vi "Expand FIFO Type Def Release.vi"(7 "Control Refnum":refnum<vi>, 8 "error in (no error)":errorcluster, 10 "Array":refnum<vi>[](array[refnum]), 11 "Cluster in":refnum<vi>) -> (0 "error out":errorcluster)   [LabVIEW 2014, in "Initialization and IO Node Scripting.lvlib"]
uses:
  Initialization and IO Node Scripting.lvlib
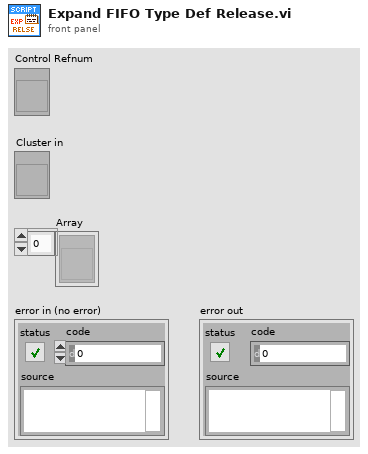
[diagram p1: front panel]
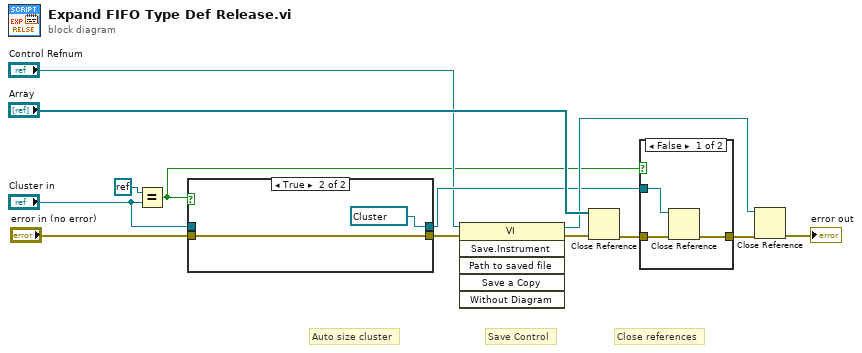
[diagram p0: block diagram]
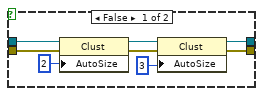
[diagram p3: hidden frame]
diagram:
  # "Auto size cluster"
  # "Save Control"
  # "Close references"
  n1 = Equal?(x=refnum<k0> refnum, y="Cluster in") -> (x = y?=w1:bool)
  n2 = case shown="True" w1 {
    tunnel: "error in (no error)" -> [w21 w23]
    tunnel: [w16 w23] -> w6
    tunnel: [w15 refnum<vi> refnum ("Cluster in")] -> w5
    tunnel: "Cluster in" -> [w14 _]
    frame False {
      n3 = property class="Clust"(reference=w14, error in=w21, "AutoSize"=u32 2 ("Auto Sizing")) -> (reference out=w19:refnum<vi>, error out=w18:errorcluster)
      n4 = property class="Clust"(reference=w19, error in=w18, "AutoSize"=u32 3 ("Auto Sizing")) -> (reference out=w15:refnum<vi>, error out=w16:errorcluster)
    }
    frame True {
    }
  }
  n5 = invoke class="VI" method="Save.Instrument"(reference="Control Refnum", error in=w6) -> (reference out=w10:refnum<vi>, error out=w7:errorcluster)  [unwired: 4 in, 4 out]
  n6 = Close Reference(reference="Array", error in (no error)=w7) -> (error out=w8:errorcluster)
  n7 = case shown="False" w1 {
    tunnel: [w26 w27] -> w9
    tunnel: w8 -> [w25 w27]
    tunnel: w5 -> [w24 _]
    frame False {
      n8 = Close Reference(reference=w24, error in (no error)=w25) -> (error out=w26:errorcluster)
    }
    frame True {
    }
  }
  n9 = Close Reference(reference=w10, error in (no error)=w9) -> (error out=→"error out":errorcluster)
